vi "Test 1.vi"(8 "error in (no error)":errorcluster, 11 "Test Case In":refnum<class "Tests.lvclass">) -> (0 "error out":errorcluster, 3 "Test Case Out":refnum<class "Tests.lvclass">)   [LabVIEW 2020, in "Tests.lvclass"]
uses:
  Tests.lvclass
  C:/Program Files (x86)/National Instruments/LabVIEW 2020/vi.lib/Astemes/LUnit/Test Case.lvclass
  <vilib>/Astemes/LUnit/Test Case.lvclass/Test Case.ctl
  <vilib>/Astemes/LUnit/Append Fail Result.vi
  <vilib>/Astemes/LUnit/Append Pass Result.vi
  <vilib>/Astemes/LUnit/Run In UI.vi
  <vilib>/Utility/error.llb/Clear Errors.vi
  Tests.lvclass/Tests.ctl
  Proto/Proto.lvclass
  <vilib>/Astemes/LUnit/Test Case.lvclass
  C:/Program Files (x86)/National Instruments/LabVIEW 2020/vi.lib/Astemes/LUnit/LUnit Runnable.lvclass
  C:/git/aoc-2023/Day 24_24/Tests/Tests.lvclass
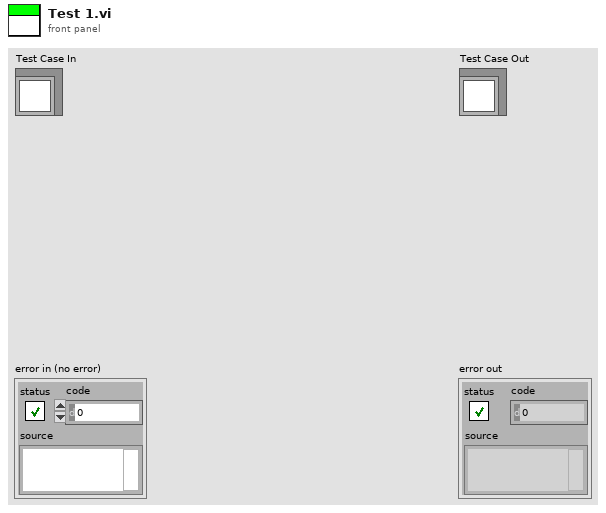
[diagram p1: front panel]
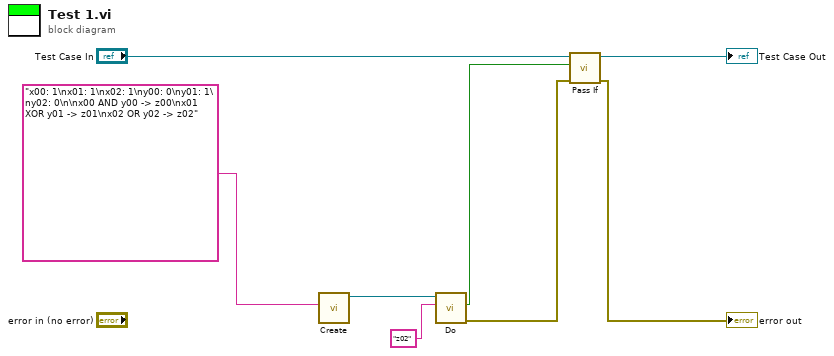
[diagram p0: block diagram]
diagram:
  n1 = call "Create.vi"("Input"="x00: 1\nx01: 1\nx02: 1\ny00: 0\ny01: 1\ny02: 0\n\nx00 AND y00 -> z00\nx01 XOR y01 -> z01\nx02 OR y02 -> z02") -> ("Proto"=w4:refnum<class "Proto.lvclass">)  [unwired: 10 in]
  n2 = call "Do.vi"("Key"="z02", "Proto in"=w4) -> ("error out"=w5:errorcluster, "Value"=w1:bool)  [unwired: 7 in, 1 out]
  n3 = call <vilib>:"Pass If.vi"("error in (no error)"=w5, "Pass?"=w1, "LUnit Test Case In"="Test Case In") -> ("error out"=→"error out":errorcluster, "LUnit Test Case Out"=→"Test Case Out":refnum<class "Tests.lvclass">)  [unwired: 7 in]
